vi "Microphone_example.vi"() -> ()   [LabVIEW 2022 SP3]
doc: "This VI illustrates how to acquire sound samples continuously from a specified device. It requires the use of a microphone attached to the sound card. You can specify the number of samples to acquire, sample rate, number of channels and a bit rate per sample. The VI also plots the raw data as the acquisition is made."
uses:
  <vilib>/sound2/lvsound2.llb/Sampling Mode.ctl
  <vilib>/sound2/lvsound2.llb/Sound Input Read (DBL).vi
  <vilib>/measure/mascope.llb/Amplitude and Levels N chan.vi
  <resource>/lvsound2.dll
  <vilib>/measure/NI_MAPro.lvlib
panel:
  in  "Select your device":u32(knob) scale=0.0..3.0
  in  "Begin Measuring":bool
  out "devName":string
  out "Raw Data":waveform(dbl)[](graph)
  in  "Stop":bool
  # "1. Select your input device by using the knob\n2. Once the appropriate device is selected, press Begin\n3. Exit the program with the STOP button"
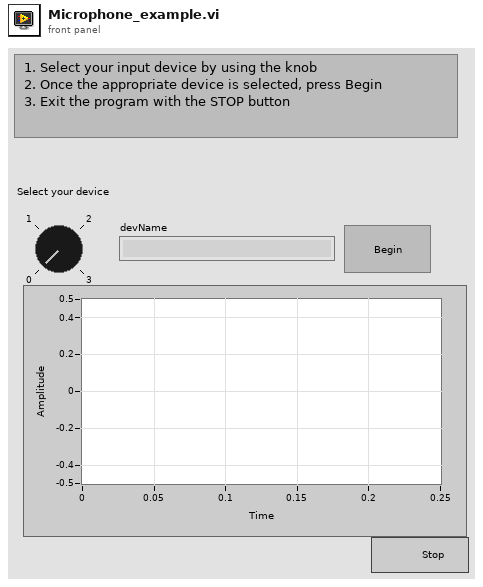
[diagram p1: front panel]
types:
  T1 = typedef "Sampling Mode.ctl" = i32
  T2 = typedef "Sound Input Task ID.ctl" = u32
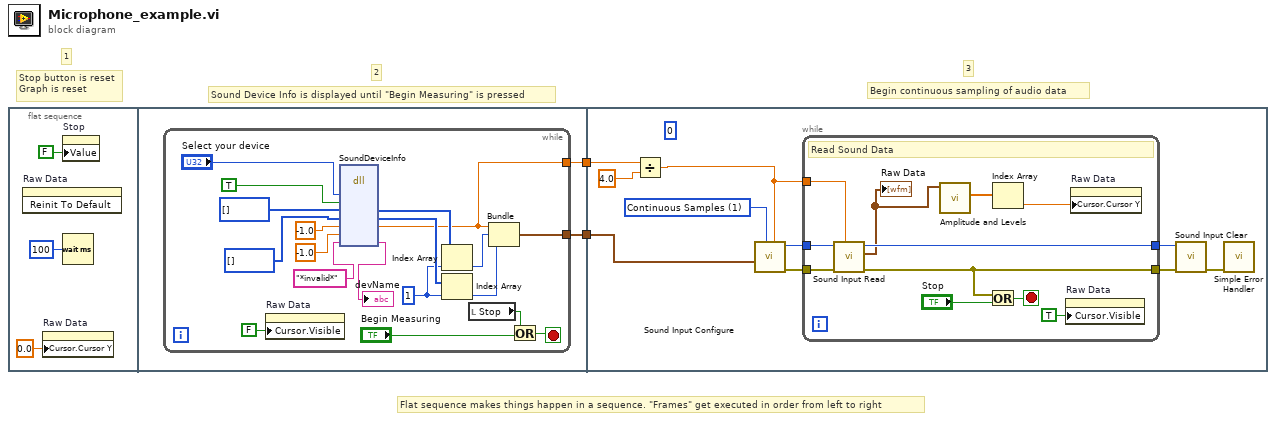
[diagram p0: block diagram]
diagram:
  # "3"
  # "2"
  # "1"
  # "Begin continuous sampling of audio data"
  # "Sound Device Info is displayed until \"Begin Measuring\" is pressed"
  # "Flat sequence makes things happen in a sequence. \"Frames\" get executed in order from left to right"
  # "Stop button is reset\nGraph is reset"
  n1 = flat-sequence {
    tunnel: [w7] -> w2
    tunnel: [w6] -> w1
    tunnel: w2 -> [w30]
    tunnel: w1 -> [w28]
    frame #0 {
      n2 = invoke on="Raw Data" class="WFGraph (strict)" method="Reinit To Default"() -> ()  [unwired: 3 in, 3 out]
      n3 = property on="Raw Data" class="WFGraph (strict)"("Cursor.Cursor Y"=0.0 ("Cursor.Cursor Position:Cursor Y")) -> ()  [unwired: 2 in, 2 out]
      n4 = property on="Stop" class="Bool (strict)"("Value"=FALSE ("Stop")) -> ()  [unwired: 2 in, 2 out]
      n5 = Wait (ms)(milliseconds to wait=u32 100) -> ()  [unwired: 1 out]
    }
    frame #1 {
      n6 = while {
        tunnel: [w14] -> w7
        tunnel: [w13] -> w6
        stop <- w12 stop-if-true
        w9 = 1 ("index")
        n7 = property on="Raw Data" class="WFGraph (strict)"("Cursor.Visible"=FALSE) -> ()  [unwired: 2 in, 2 out]
        n8 = dll-call lib="C:/Program Files/National Instruments/LabVIEW 2022/resource/lvsound2.*" fn="SoundDeviceInfo"("device"="Select your device", "isInput"=TRUE, "channels"=i32[] [] ("numChannels"), "depths"=i32[] [] ("sampleDepths"), "minFreq"=-1.0, "maxFreq"=-1.0, "devName"="*invalid*") -> ("channels"=w17:i32[], "depths"=w18:i32[], "minFreq"=w13:dbl, "devName"=→"devName":string)  [unwired: 5 in, 4 out]
        n9 = Index Array(array=w17, index=w9) -> (element=w16:i32)
        n10 = Index Array(array=w18, index=w9) -> (element=w15:i32)
        n11 = local read "Stop"() -> (w11:bool)
        n12 = Bundle("minFreq"=w13, w16, w15) -> (w14:cluster{"minFreq":dbl, i32, i32})  [unwired: 1 in]
        n13 = Or(x=w11, y="Begin Measuring") -> (x .or. y?=w12:bool)
      }
    }
    frame #2 {
      (unwired) 0
      w31 = T1 1 items=["Finite Samples", "Continuous Samples"] ("sample mode")
      n14 = Divide(x=w28, y=4.0) -> (x/y=w27:dbl)
      n15 = call <vilib>:"Sound Input Configure.vi"("number of samples/ch"=w27, "sample mode"=w31, "sound format"=w30) -> ("error out"=w32:errorcluster, "task ID"=w33:T2)  [unwired: 7 in]
      n16 = while {
        tunnel: w33 -> [w46]
        tunnel: [w45] -> w34
        tunnel: w27 -> [w44]
        tunnel: w32 -> [w47]
        tunnel: [w41] -> w35
        stop <- w42 stop-if-true
        # "Read Sound Data"
        n17 = call-poly <vilib>:"Sound Input Read.vi"("number of samples/ch"=w44, "error in (no error)"=w47, "task ID"=w46) -> ("error out"=w41:errorcluster, "data"=w40:waveform(dbl)[], "task ID out"=w45:T2)  [unwired: 6 in]
        "Raw Data" <- w40
        n18 = call-poly <vilib>:"Amplitude and Levels.vi"("signal(s) in"=w40) -> ("high state level"=w39:dbl[])  [unwired: 7 in, 3 out]
        n19 = Or(x=w41, y="Stop") -> (x .or. y?=w42:bool)
        n20 = Index Array "Index Array"(array=w39) -> (element=w38:dbl)  [unwired: 1 in]
        n21 = property on="Raw Data" class="WFGraph (strict)"("Cursor.Visible"=TRUE) -> ()  [unwired: 2 in, 2 out]
        n22 = property on="Raw Data" class="WFGraph (strict)"("Cursor.Cursor Y"=w38) -> ()  [unwired: 2 in, 2 out]
      }
      n23 = call <vilib>:"Sound Input Clear.vi"("error in (no error)"=w35, "task ID"=w34) -> ("error out"=w36:errorcluster)  [unwired: 9 in]
      n24 = call <vilib>:"Simple Error Handler.vi"("error in (no error)"=w36) -> ()  [unwired: 4 in, 5 out]
    }
  }
